vi "Read System Data.vi"(8 "Error In":errorcluster, 10 "Modbus ID":string, 11 "VISA resource name":refnum<visa-resource-name>) -> (0 "Error Out":errorcluster, 2 "AFV-P System Data":T1 {"Freq Lo Limit" format="%#.1f Hz"; "Freq Hi Limit" format="%#.1f Hz"; "Volt Lo Limit" format="%.1f V"; "Volt Hi Limit" format="%.1f V"; "DC Volt Lo Limit" format="%.1f V"; "DC Volt Hi Limit" format="%.1f V"}, 3 "VISA resource name out":refnum<visa-resource-name>)   [LabVIEW 2013]
panel:
  out "Data":string
  # "."
  # "."
  # "."
  # "."
  # "."
  # "."
  # "."
  # "."
  # "."
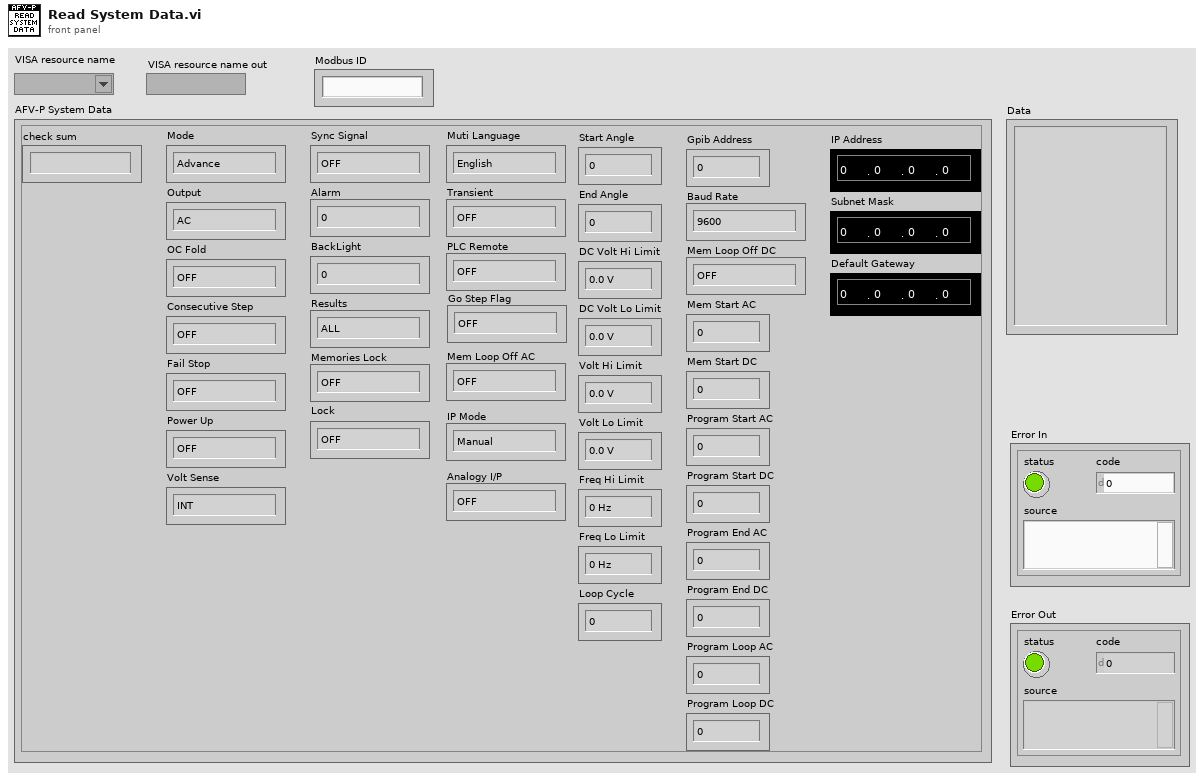
[diagram p1: front panel]
types:
  T1 = cluster{"check sum":string, "Mode":enum16{"Advance", "Basic"}, "Output":enum16{"AC", "DC"}, "OC Fold":enum16{"OFF", "ON"}, "Consecutive Step":enum16{"OFF", "ON"}, "Fail Stop":enum16{"OFF", "ON"}, "Power Up":enum16{"OFF", "ON", "LAST"}, "Volt Sense":enum16{"INT", "EXT"}, "Sync Signal":enum16{"OFF", "ON", "EVENT"}, "Alarm":enum16{"0", "1", "2", "3", "4", "5", "6", "7", "8", "9"}, "BackLight":enum16{"0", "1", "2", "3", "4", "5", "6", "7", "8", "9"}, "Results":enum16{"ALL", "P/F", "LAST"}, "Memories Lock":enum16{"OFF", "ON"}, "Lock":enum16{"OFF", "ON"}, "Muti Language":enum16{"English", "繁體中文", "簡體中文", "日文"}, "Transient":enum16{"OFF", "ON"}, "PLC Remote":enum16{"OFF", "ON"}, "Go Step Flag":enum16{"OFF", "ON"}, "Mem Loop Off AC":enum16{"OFF", "ON"}, "IP Mode":enum16{"Manual", "Auto"}, "Analogy I/P":enum16{"OFF", "ON"}, "Start Angle":u16, "End Angle":u16, "DC Volt Hi Limit":dbl, "DC Volt Lo Limit":dbl, "Volt Hi Limit":dbl, "Volt Lo Limit":dbl, "Freq Hi Limit":dbl, "Freq Lo Limit":dbl, "Loop Cycle":u16, "Gpib Address":u8, "Baud Rate":enum16{"9600", "19200", "38400", "57600", "115200"}, "Mem Loop Off DC":enum16{"OFF", "ON"}, "Mem Start AC":u8, "Mem Start DC":u8, "Program Start AC":u16, "Program Start DC":u16, "Program End AC":u16, "Program End DC":u16, "Program Loop AC":u16, "Program Loop DC":u16, "IP Address":cluster{"IP 0":u8, "IP 1":u8, "IP 2":u8, "IP 3":u8}, "Subnet Mask":cluster{"IP 0":u8, "IP 1":u8, "IP 2":u8, "IP 3":u8}, "Default Gateway":cluster{"IP 0":u8, "IP 1":u8, "IP 2":u8, "IP 3":u8}}
  T2 = cluster{"ID":string, "Function Code":string, "Length (High)":string, "Length (Low)":string, "Start Address (High)":string, "Start Address (Middle High)":string, "Start Address (Middle Low)":string, "Start Address (Low)":string, "Data":string}
  T3 = cluster{"Length (High)":string, "Length (Low)":string, "Start Address (High)":string, "Start Address (Middle High)":string, "Start Address (Middle Low)":string, "Start Address (Low)":string}
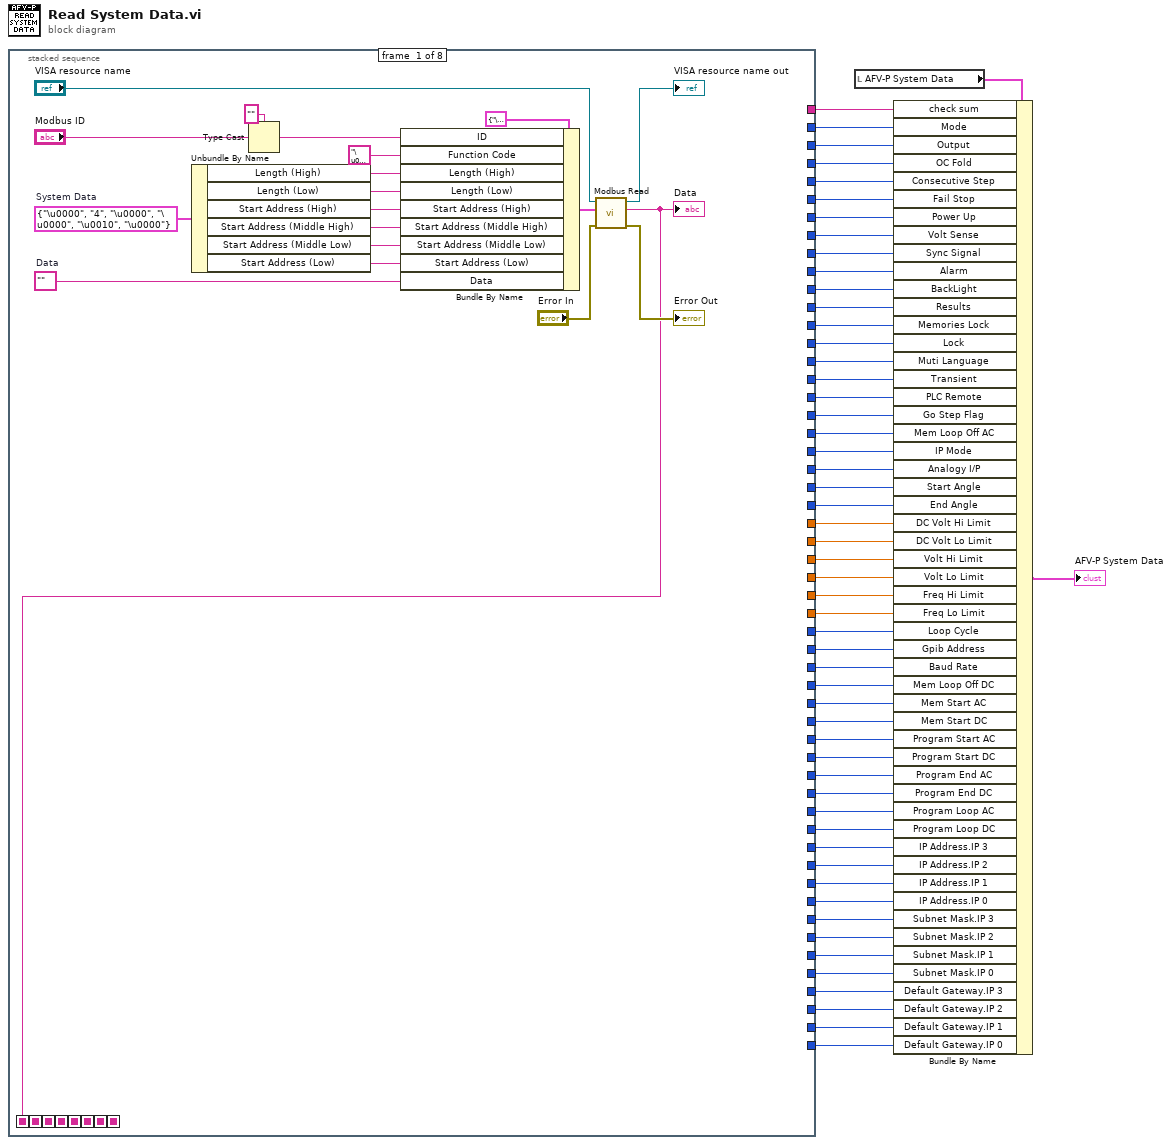
[diagram p0: block diagram]
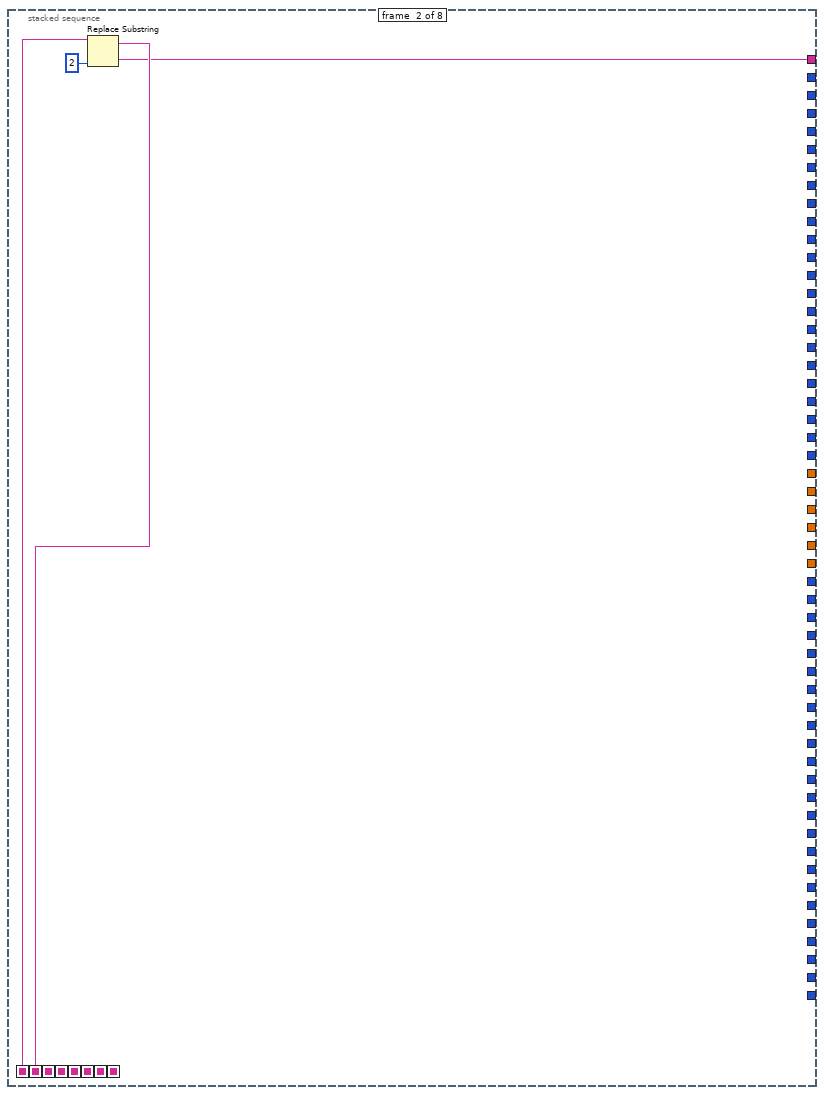
[diagram p2: hidden frame]
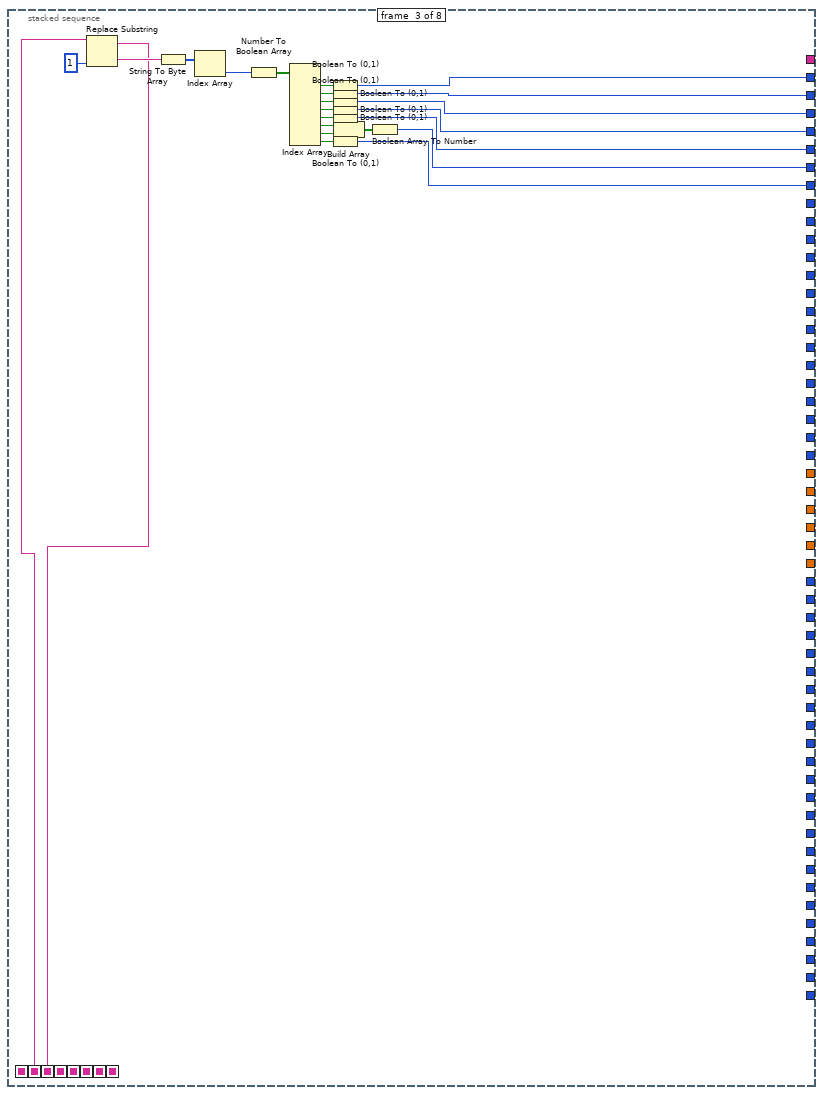
[diagram p3: hidden frame]
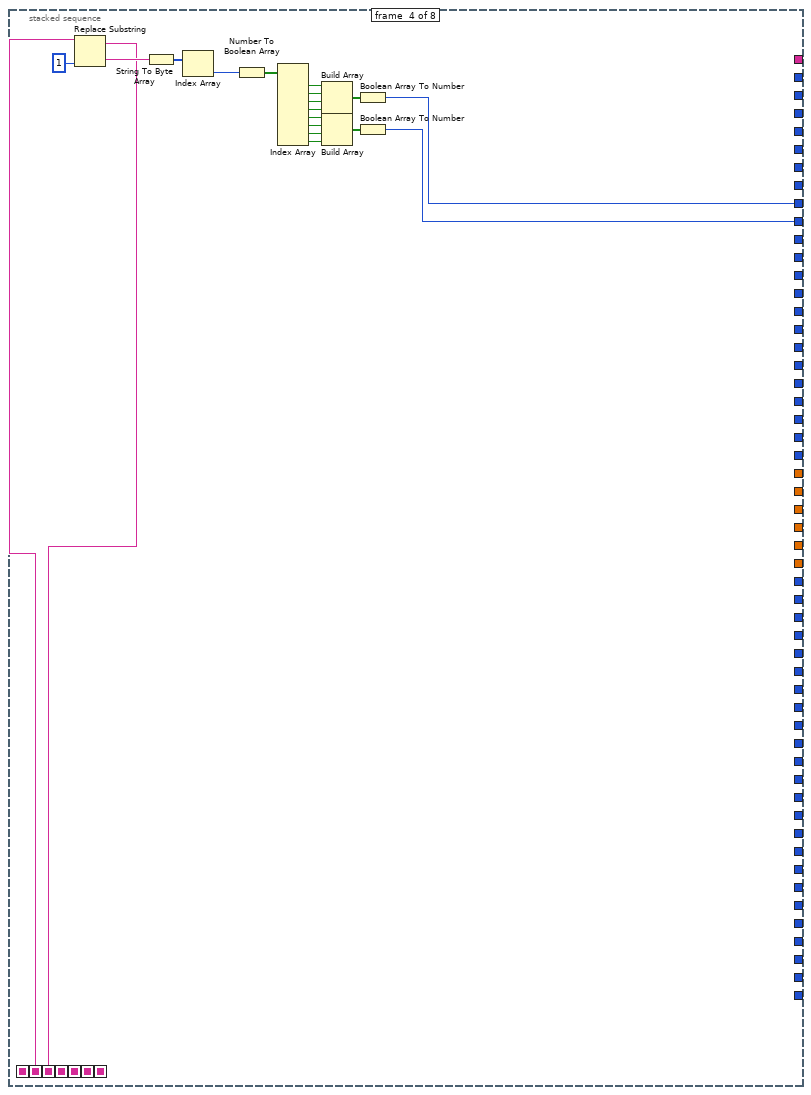
[diagram p4: hidden frame]
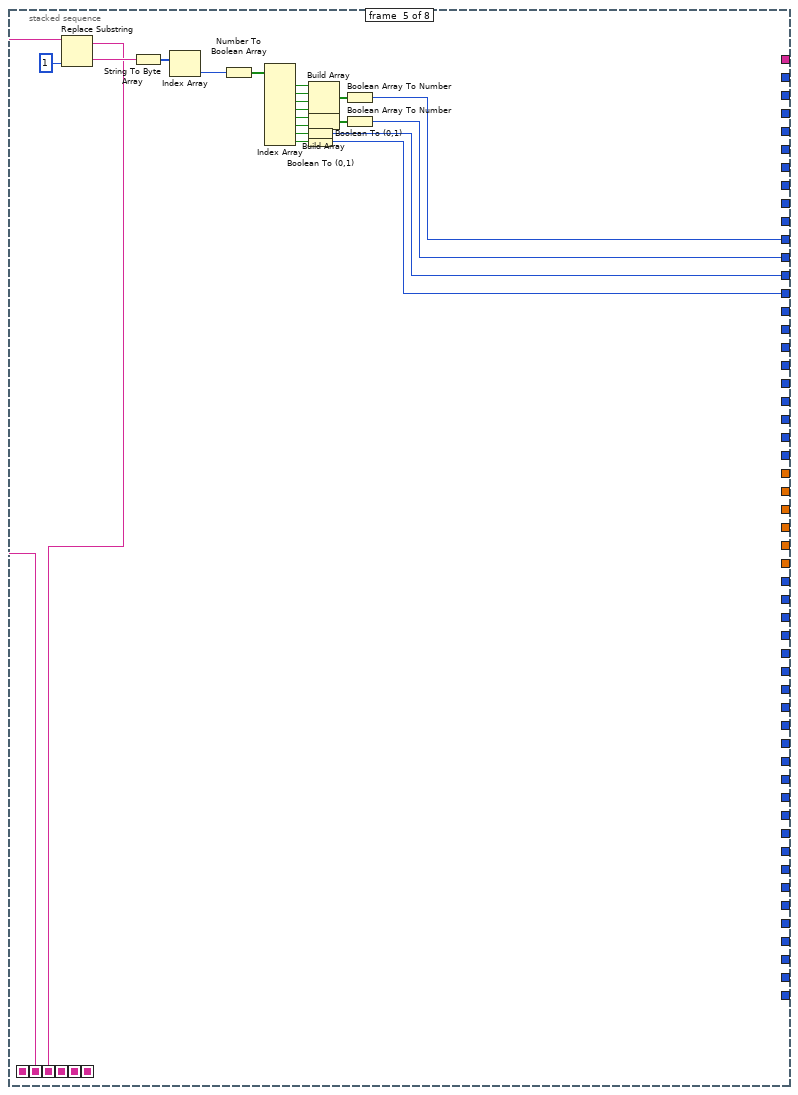
[diagram p5: hidden frame]
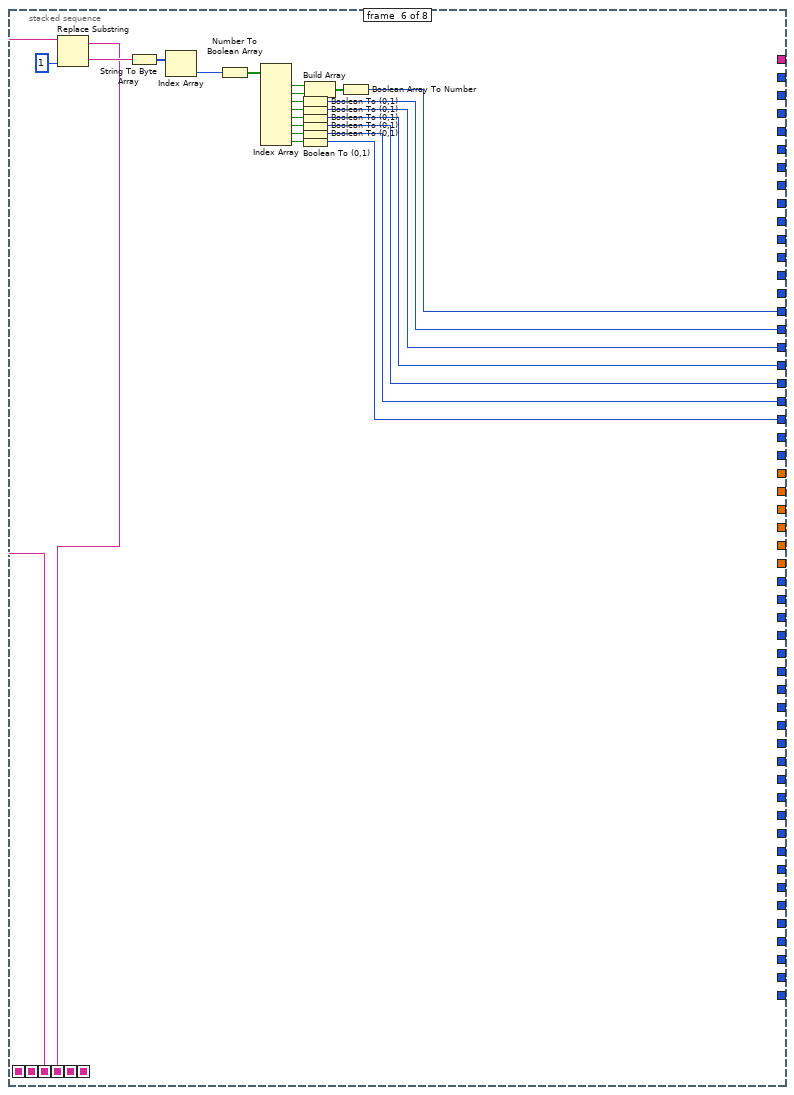
[diagram p6: hidden frame]
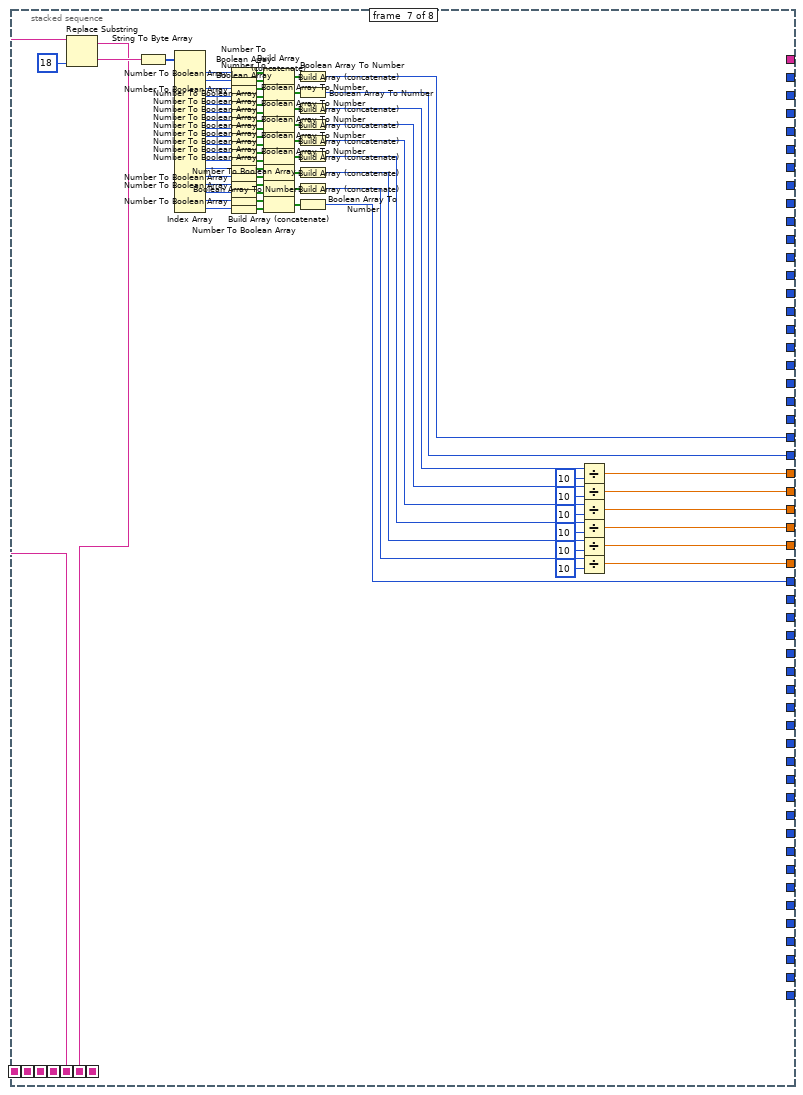
[diagram p7: hidden frame]
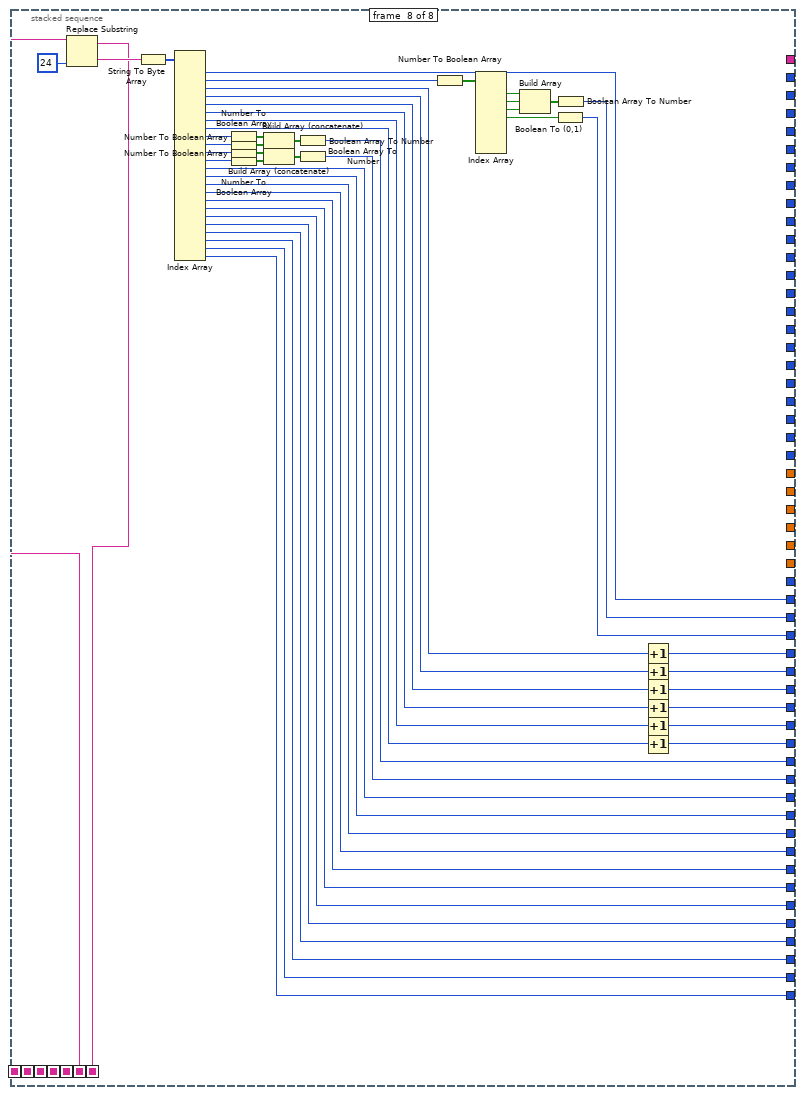
[diagram p8: hidden frame]
diagram:
  n1 = stacked-sequence {
    seq-local: [w63 _ _ _ _ _ _ _] -> [_ w77 _ _ _ _ _ _]
    seq-local: [_ w76 _ _ _ _ _ _] -> [_ _ w86 _ _ _ _ _]
    seq-local: [_ _ w87 _ _ _ _ _] -> [_ _ _ w104 _ _ _ _]
    seq-local: [_ _ _ w105 _ _ _ _] -> [_ _ _ _ w127 _ _ _]
    seq-local: [_ _ _ _ w128 _ _ _] -> [_ _ _ _ _ w155 _ _]
    seq-local: [_ _ _ _ _ w156 _ _] -> [_ _ _ _ _ _ w231 _]
    seq-local: [_ _ _ _ _ _ w232 _] -> [_ _ _ _ _ _ _ w282]
    seq-local: [_ _ _ _ _ _ _ w283] -> [_ _ _ _ _ _ _ _]
    tunnel: [_ w75 _ _ _ _ _ _] -> w55
    tunnel: [_ _ w85 _ _ _ _ _] -> w54
    tunnel: [_ _ w84 _ _ _ _ _] -> w53
    tunnel: [_ _ w83 _ _ _ _ _] -> w52
    tunnel: [_ _ w82 _ _ _ _ _] -> w51
    tunnel: [_ _ w81 _ _ _ _ _] -> w50
    tunnel: [_ _ w80 _ _ _ _ _] -> w49
    tunnel: [_ _ w79 _ _ _ _ _] -> w48
    tunnel: [_ _ _ w103 _ _ _ _] -> w47
    tunnel: [_ _ _ w102 _ _ _ _] -> w46
    tunnel: [_ _ _ _ w124 _ _ _] -> w45
    tunnel: [_ _ _ _ w123 _ _ _] -> w44
    tunnel: [_ _ _ _ w122 _ _ _] -> w43
    tunnel: [_ _ _ _ w121 _ _ _] -> w42
    tunnel: [_ _ _ _ _ w152 _ _] -> w41
    tunnel: [_ _ _ _ _ w151 _ _] -> w40
    tunnel: [_ _ _ _ _ w150 _ _] -> w39
    tunnel: [_ _ _ _ _ w148 _ _] -> w38
    tunnel: [_ _ _ _ _ _ w195 _] -> w37
    tunnel: [_ _ _ _ _ _ w194 _] -> w36
    tunnel: [_ _ _ _ _ _ w191 _] -> w35
    tunnel: [_ _ _ _ _ _ w188 _] -> w34
    tunnel: [_ _ _ _ _ _ w187 _] -> w33
    tunnel: [_ _ _ _ _ _ w175 _] -> w32
    tunnel: [_ _ _ _ _ _ _ w268] -> w31
    tunnel: [_ _ _ _ _ _ _ w266] -> w30
    tunnel: [_ _ _ _ _ _ _ w263] -> w10
    tunnel: [_ _ _ _ _ _ _ w275] -> w8
    tunnel: [_ _ _ _ _ _ _ w274] -> w7
    tunnel: [_ _ _ _ _ _ _ w262] -> w6
    tunnel: [_ _ _ _ _ _ w186 _] -> w29
    tunnel: [_ _ _ _ _ _ w168 _] -> w28
    tunnel: [_ _ _ _ _ _ w167 _] -> w27
    tunnel: [_ _ _ _ _ w144 _ _] -> w26
    tunnel: [_ _ _ _ _ w143 _ _] -> w25
    tunnel: [_ _ _ _ _ w142 _ _] -> w24
    tunnel: [_ _ _ _ _ _ _ w249] -> w23
    tunnel: [_ _ _ _ _ _ _ w248] -> w22
    tunnel: [_ _ _ _ _ _ _ w247] -> w21
    tunnel: [_ _ _ _ _ _ _ w246] -> w20
    tunnel: [_ _ _ _ _ _ _ w245] -> w19
    tunnel: [_ _ _ _ _ _ _ w244] -> w18
    tunnel: [_ _ _ _ _ _ _ w243] -> w17
    tunnel: [_ _ _ _ _ _ _ w242] -> w16
    tunnel: [_ _ _ _ _ _ _ w241] -> w15
    tunnel: [_ _ _ _ _ _ _ w240] -> w14
    tunnel: [_ _ _ _ _ _ _ w239] -> w13
    tunnel: [_ _ _ _ _ _ _ w238] -> w12
    tunnel: [_ _ _ _ _ _ _ w264] -> w11
    tunnel: [_ _ _ _ _ _ _ w260] -> w9
    tunnel: [_ _ _ _ _ _ _ w236] -> w5
    tunnel: [_ _ _ _ _ _ _ w237] -> w4
    tunnel: [_ _ _ _ _ _ _ w254] -> w3
    frame #0 {
      w62 = T3 {"Length (High)"="\u0000", "Length (Low)"="4", "Start Address (High)"="\u0000", "Start Address (Middle High)"="\u0000", "Start Address (Middle Low)"="\u0010", "Start Address (Low)"="\u0000"}  # System Data
      w70 = ""  # Data
      n2 = Unbundle By Name(w62) -> ("Length (High)"=w69:string, "Length (Low)"=w68:string, "Start Address (High)"=w67:string, "Start Address (Middle High)"=w66:string, "Start Address (Middle Low)"=w65:string, "Start Address (Low)"=w64:string)
      n3 = Type Cast(type="" ("Binary Data (Hex) 3"), x="Modbus ID") -> (*(type *) &x=w56:string)
      n4 = Bundle By Name(cluster=T2 {"ID"="\u0000", "Function Code"="\u0000", "Length (High)"="\u0000", "Length (Low)"="\u0000", "Start Address (High)"="\u0000", "Start Address (Middle High)"="\u0000", "Start Address (Middle Low)"="\u0000", "Start Address (Low)"="\u0000", "Data"=""} ("Write Buffer"), "ID"=w56, "Function Code"="\u0003", "Length (High)"=w69, "Length (Low)"=w68, "Start Address (High)"=w67, "Start Address (Middle High)"=w66, "Start Address (Middle Low)"=w65, "Start Address (Low)"=w64, "Data"=w70) -> (w73:T2)
      n5 = call "Modbus Read.vi"("Error In"="Error In", "Write Buffer"=w73, "VISA resource name"="VISA resource name") -> ("Error Out"=→"Error Out":errorcluster, "Read Data"=w63:string, "VISA resource name out"=→"VISA resource name out":refnum<visa-resource-name>)  [unwired: 6 in]
      "Data" <- w63
    }
    frame #1 {
      n6 = Replace Substring(2:2 ("length (len. of substring)"), 5:w77) -> (0:w75:string, 1:w76:string)  [unwired: 2 in]
    }
    frame #2 {
      n7 = Replace Substring(2:1 ("length (len. of substring)"), 5:w86) -> (0:w88:string, 1:w87:string)  [unwired: 2 in]
      n8 = String To Byte Array(string=w88) -> (unsigned byte array=w89:u8[])
      n9 = Index Array(array=w89) -> (element=w90:u8)  [unwired: 1 in]
      n10 = Number To Boolean Array(number=w90) -> (Boolean array=w91:bool[])
      n11 = Index Array(array=w91) -> (element #1=w92:bool, element #2=w93:bool, element #3=w94:bool, element #4=w95:bool, element #5=w96:bool, element #6=w97:bool, element #7=w98:bool, element #8=w100:bool)  [unwired: 8 in]
      n12 = Boolean To (0,1)(Boolean=w92) -> (0, 1=w85:i16)
      n13 = Boolean To (0,1)(Boolean=w93) -> (0, 1=w84:i16)
      n14 = Boolean To (0,1)(Boolean=w94) -> (0, 1=w83:i16)
      n15 = Boolean To (0,1)(Boolean=w95) -> (0, 1=w82:i16)
      n16 = Boolean To (0,1)(Boolean=w96) -> (0, 1=w81:i16)
      n17 = Boolean To (0,1)(Boolean=w100) -> (0, 1=w79:i16)
      n18 = Build Array(w97, w98) -> (w99:bool[])
      n19 = Boolean Array To Number(Boolean array=w99) -> (number=w80:u32)
    }
    frame #3 {
      n20 = Replace Substring(2:1 ("length (len. of substring)"), 5:w104) -> (0:w117:string, 1:w105:string)  [unwired: 2 in]
      n21 = String To Byte Array(string=w117) -> (unsigned byte array=w118:u8[])
      n22 = Index Array(array=w118) -> (element=w119:u8)  [unwired: 1 in]
      n23 = Number To Boolean Array(number=w119) -> (Boolean array=w106:bool[])
      n24 = Index Array(array=w106) -> (element #1=w107:bool, element #2=w108:bool, element #3=w109:bool, element #4=w110:bool, element #5=w112:bool, element #6=w113:bool, element #7=w114:bool, element #8=w115:bool)  [unwired: 8 in]
      n25 = Build Array(w107, w108, w109, w110) -> (w111:bool[])
      n26 = Build Array(w112, w113, w114, w115) -> (w116:bool[])
      n27 = Boolean Array To Number(Boolean array=w111) -> (number=w103:u32)
      n28 = Boolean Array To Number(Boolean array=w116) -> (number=w102:u32)
    }
    frame #4 {
      n29 = Replace Substring(2:1 ("length (len. of substring)"), 5:w127) -> (0:w138:string, 1:w128:string)  [unwired: 2 in]
      n30 = String To Byte Array(string=w138) -> (unsigned byte array=w139:u8[])
      n31 = Index Array(array=w139) -> (element=w140:u8)  [unwired: 1 in]
      n32 = Number To Boolean Array(number=w140) -> (Boolean array=w129:bool[])
      n33 = Index Array(array=w129) -> (element #1=w130:bool, element #2=w131:bool, element #3=w132:bool, element #4=w133:bool, element #5=w135:bool, element #6=w136:bool, element #7=w126:bool, element #8=w125:bool)  [unwired: 8 in]
      n34 = Boolean To (0,1)(Boolean=w126) -> (0, 1=w122:i16)
      n35 = Boolean To (0,1)(Boolean=w125) -> (0, 1=w121:i16)
      n36 = Build Array(w130, w131, w132, w133) -> (w134:bool[])
      n37 = Build Array(w135, w136) -> (w137:bool[])
      n38 = Boolean Array To Number(Boolean array=w134) -> (number=w124:u32)
      n39 = Boolean Array To Number(Boolean array=w137) -> (number=w123:u32)
    }
    frame #5 {
      n40 = Replace Substring(2:1 ("length (len. of substring)"), 5:w155) -> (0:w161:string, 1:w156:string)  [unwired: 2 in]
      n41 = String To Byte Array(string=w161) -> (unsigned byte array=w162:u8[])
      n42 = Index Array(array=w162) -> (element=w163:u8)  [unwired: 1 in]
      n43 = Number To Boolean Array(number=w163) -> (Boolean array=w157:bool[])
      n44 = Index Array(array=w157) -> (element #1=w158:bool, element #2=w159:bool, element #3=w154:bool, element #4=w153:bool, element #5=w149:bool, element #6=w146:bool, element #7=w145:bool, element #8=w147:bool)  [unwired: 8 in]
      n45 = Boolean To (0,1)(Boolean=w154) -> (0, 1=w151:i16)
      n46 = Boolean To (0,1)(Boolean=w153) -> (0, 1=w150:i16)
      n47 = Boolean To (0,1)(Boolean=w149) -> (0, 1=w148:i16)
      n48 = Boolean To (0,1)(Boolean=w146) -> (0, 1=w144:i16)
      n49 = Boolean To (0,1)(Boolean=w145) -> (0, 1=w143:i16)
      n50 = Boolean To (0,1)(Boolean=w147) -> (0, 1=w142:i16)
      n51 = Build Array(w158, w159) -> (w160:bool[])
      n52 = Boolean Array To Number(Boolean array=w160) -> (number=w152:u32)
    }
    frame #6 {
      n53 = Replace Substring(2:18 ("length (len. of substring)"), 5:w231) -> (0:w233:string, 1:w232:string)  [unwired: 2 in]
      n54 = String To Byte Array(string=w233) -> (unsigned byte array=w234:u8[])
      n55 = Index Array(array=w234) -> (element #1=w227:u8, element #2=w226:u8, element #3=w222:u8, element #4=w221:u8, element #5=w214:u8, element #6=w213:u8, element #7=w212:u8, element #8=w211:u8, element #9=w204:u8, element #10=w203:u8, element #11=w202:u8, element #12=w201:u8, element #13=w197:u8, element #14=w196:u8, element #15=w179:u8, element #16=w178:u8, element #17=w177:u8, element #18=w176:u8)  [unwired: 18 in]
      n56 = Number To Boolean Array(number=w227) -> (Boolean array=w229:bool[])
      n57 = Number To Boolean Array(number=w226) -> (Boolean array=w230:bool[])
      n58 = Number To Boolean Array(number=w222) -> (Boolean array=w224:bool[])
      n59 = Number To Boolean Array(number=w221) -> (Boolean array=w223:bool[])
      n60 = Number To Boolean Array(number=w214) -> (Boolean array=w216:bool[])
      n61 = Number To Boolean Array(number=w213) -> (Boolean array=w215:bool[])
      n62 = Number To Boolean Array(number=w212) -> (Boolean array=w219:bool[])
      n63 = Number To Boolean Array(number=w211) -> (Boolean array=w220:bool[])
      n64 = Number To Boolean Array(number=w204) -> (Boolean array=w209:bool[])
      n65 = Number To Boolean Array(number=w203) -> (Boolean array=w210:bool[])
      n66 = Number To Boolean Array(number=w202) -> (Boolean array=w206:bool[])
      n67 = Number To Boolean Array(number=w201) -> (Boolean array=w205:bool[])
      n68 = Number To Boolean Array(number=w197) -> (Boolean array=w199:bool[])
      n69 = Number To Boolean Array(number=w196) -> (Boolean array=w200:bool[])
      n70 = Number To Boolean Array(number=w179) -> (Boolean array=w181:bool[])
      n71 = Number To Boolean Array(number=w178) -> (Boolean array=w182:bool[])
      n72 = Number To Boolean Array(number=w177) -> (Boolean array=w184:bool[])
      n73 = Number To Boolean Array(number=w176) -> (Boolean array=w183:bool[])
      n74 = Build Array (concatenate)(w229, w230) -> (w228:bool[])
      n75 = Build Array (concatenate)(w224, w223) -> (w225:bool[])
      n76 = Build Array (concatenate)(w216, w215) -> (w217:bool[])
      n77 = Build Array (concatenate)(w219, w220) -> (w218:bool[])
      n78 = Build Array (concatenate)(w209, w210) -> (w208:bool[])
      n79 = Build Array (concatenate)(w206, w205) -> (w207:bool[])
      n80 = Build Array (concatenate)(w199, w200) -> (w198:bool[])
      n81 = Build Array (concatenate)(w181, w182) -> (w180:bool[])
      n82 = Build Array (concatenate)(w184, w183) -> (w185:bool[])
      n83 = Boolean Array To Number(Boolean array=w228) -> (number=w186:u32)
      n84 = Boolean Array To Number(Boolean array=w225) -> (number=w195:u32)
      n85 = Boolean Array To Number(Boolean array=w217) -> (number=w166:u32)
      n86 = Boolean Array To Number(Boolean array=w218) -> (number=w165:u32)
      n87 = Boolean Array To Number(Boolean array=w208) -> (number=w171:u32)
      n88 = Boolean Array To Number(Boolean array=w207) -> (number=w172:u32)
      n89 = Boolean Array To Number(Boolean array=w198) -> (number=w173:u32)
      n90 = Boolean Array To Number(Boolean array=w180) -> (number=w174:u32)
      n91 = Boolean Array To Number(Boolean array=w185) -> (number=w175:u32)
      n92 = Divide(x=w166, y=u32 10) -> (x/y=w168:dbl)
      n93 = Divide(x=w165, y=u32 10) -> (x/y=w167:dbl)
      n94 = Divide(x=w171, y=u32 10) -> (x/y=w194:dbl)
      n95 = Divide(x=w172, y=u32 10) -> (x/y=w191:dbl)
      n96 = Divide(x=w173, y=u32 10) -> (x/y=w188:dbl)
      n97 = Divide(x=w174, y=u32 10) -> (x/y=w187:dbl)
    }
    frame #7 {
      n98 = Replace Substring(2:24 ("length (len. of substring)"), 5:w282) -> (0:w284:string, 1:w283:string)  [unwired: 2 in]
      n99 = String To Byte Array(string=w284) -> (unsigned byte array=w285:u8[])
      n100 = Index Array(array=w285) -> (element #1=w268:u8, element #2=w267:u8, element #3=w278:u8, element #4=w261:u8, element #5=w277:u8, element #6=w276:u8, element #7=w256:u8, element #8=w255:u8, element #9=w253:u8, element #10=w252:u8, element #11=w251:u8, element #12=w250:u8, element #13=w249:u8, element #14=w248:u8, element #15=w247:u8, element #16=w246:u8, element #17=w245:u8, element #18=w244:u8, element #19=w243:u8, element #20=w242:u8, element #21=w241:u8, element #22=w240:u8, element #23=w239:u8, element #24=w238:u8)  [unwired: 24 in]
      n101 = Number To Boolean Array(number=w253) -> (Boolean array=w280:bool[])
      n102 = Number To Boolean Array(number=w252) -> (Boolean array=w279:bool[])
      n103 = Number To Boolean Array(number=w251) -> (Boolean array=w258:bool[])
      n104 = Number To Boolean Array(number=w250) -> (Boolean array=w259:bool[])
      n105 = Build Array (concatenate)(w280, w279) -> (w281:bool[])
      n106 = Build Array (concatenate)(w258, w259) -> (w257:bool[])
      n107 = Boolean Array To Number(Boolean array=w281) -> (number=w237:u32)
      n108 = Boolean Array To Number(Boolean array=w257) -> (number=w236:u32)
      n109 = Number To Boolean Array(number=w267) -> (Boolean array=w269:bool[])
      n110 = Index Array(array=w269) -> (element #1=w270:bool, element #2=w271:bool, element #3=w272:bool, element #4=w265:bool)  [unwired: 8 in, 4 out]
      n111 = Build Array(w270, w271, w272) -> (w273:bool[])
      n112 = Boolean To (0,1)(Boolean=w265) -> (0, 1=w264:i16)
      n113 = Boolean Array To Number(Boolean array=w273) -> (number=w266:u32)
      n114 = Increment(x=w278) -> (x+1=w263:u8)
      n115 = Increment(x=w261) -> (x+1=w260:u8)
      n116 = Increment(x=w277) -> (x+1=w275:u8)
      n117 = Increment(x=w276) -> (x+1=w274:u8)
      n118 = Increment(x=w256) -> (x+1=w262:u8)
      n119 = Increment(x=w255) -> (x+1=w254:u8)
    }
  }
  n120 = local read "AFV-P System Data"() -> (w1:T1)
  n121 = Bundle By Name(cluster=w1, "check sum"=w55, "Mode"=w54, "Output"=w53, "OC Fold"=w52, "Consecutive Step"=w51, "Fail Stop"=w50, "Power Up"=w49, "Volt Sense"=w48, "Sync Signal"=w47, "Alarm"=w46, "BackLight"=w45, "Results"=w44, "Memories Lock"=w43, "Lock"=w42, "Muti Language"=w41, "Transient"=w40, "PLC Remote"=w39, "Go Step Flag"=w38, "Mem Loop Off AC"=w26, "IP Mode"=w25, "Analogy I/P"=w24, "Start Angle"=w29, "End Angle"=w37, "DC Volt Hi Limit"=w28, "DC Volt Lo Limit"=w27, "Volt Hi Limit"=w36, "Volt Lo Limit"=w35, "Freq Hi Limit"=w34, "Freq Lo Limit"=w33, "Loop Cycle"=w32, "Gpib Address"=w31, "Baud Rate"=w30, "Mem Loop Off DC"=w11, "Mem Start AC"=w10, "Mem Start DC"=w9, "Program Start AC"=w8, "Program Start DC"=w7, "Program End AC"=w6, "Program End DC"=w3, "Program Loop AC"=w4, "Program Loop DC"=w5, "IP Address.IP 3"=w23, "IP Address.IP 2"=w22, "IP Address.IP 1"=w21, "IP Address.IP 0"=w20, "Subnet Mask.IP 3"=w19, "Subnet Mask.IP 2"=w18, "Subnet Mask.IP 1"=w17, "Subnet Mask.IP 0"=w16, "Default Gateway.IP 3"=w15, "Default Gateway.IP 2"=w14, "Default Gateway.IP 1"=w13, "Default Gateway.IP 0"=w12) -> (→"AFV-P System Data":T1)
